vi "termometr_v2.vi"() -> ()   [LabVIEW 2023]
panel:
  in  "stop":bool
  in  "skala":bool
  out "temp. F":dbl(slide) scale=250.0..310.0 scale format="%.2g"
  out "temp. C":dbl(slide) scale=0.0..30.0 scale format="%.2g"
  # "deg C"
  # "deg F"
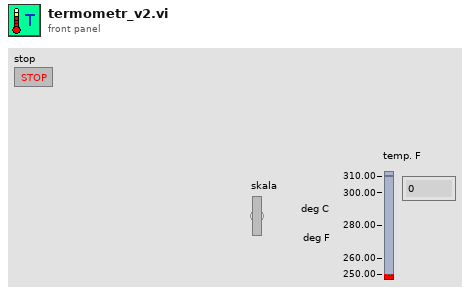
[diagram p1: front panel]
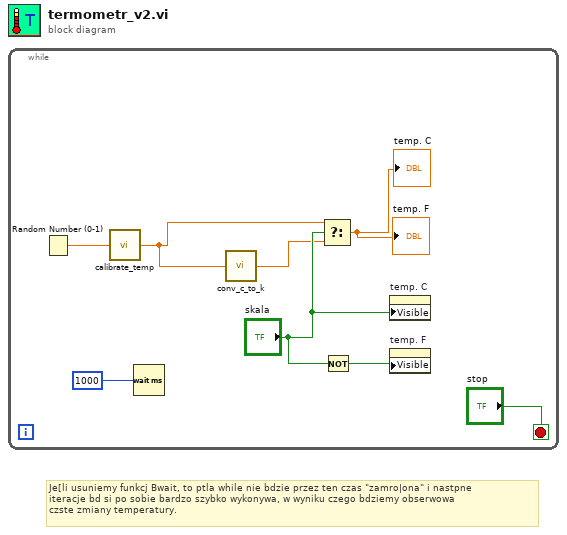
[diagram p0: block diagram]
diagram:
  # "Je[li usuniemy funkcj Bwait, to ptla while nie bdzie przez ten czas \"zamro|ona\" i nastpne\niteracje bd si po sobie bardzo szybko wykonywa, w wyniku czego bdziemy obserwowa\nczste zmiany temperatury."
  n1 = while {
    stop <- "stop" stop-if-true
    n2 = Random Number (0-1)() -> (number: 0 to 1=w4:dbl)
    n3 = call "calibrate_temp.vi"("in"=w4) -> ("out"=w2:dbl)
    n4 = Wait (ms)(milliseconds to wait=1000) -> ()  [unwired: 1 out]
    n5 = call "conv_c_to_k.vi"("deg. C"=w2) -> ("deg. K"=w1:dbl)
    n6 = Select(t=w2, s="skala", f=w1) -> (s? t:f=→"temp. C" →"temp. F":dbl)
    n7 = Not(x="skala") -> (.not. x?=w7:bool)
    n8 = property on="temp. C" class="Slide (strict)"("Visible"="skala") -> ()  [unwired: 2 in, 2 out]
    n9 = property on="temp. F" class="Slide (strict)"("Visible"=w7) -> ()  [unwired: 2 in, 2 out]
  }
